vi "FFTFiltered.vi"(0 "E4S":dbl[](array[numeric]), 1 "E3S":dbl[](array[numeric]), 4 "E2S":dbl[](array[numeric]), 5 "E1S":dbl[](array[numeric]), 6 "E6S":dbl[](array[numeric]), 7 "E5S":dbl[](array[numeric]), 11 "E8S":dbl[](array[numeric]), 12 "E7S":dbl[](array[numeric]), 14 "E9S":dbl[](array[numeric]), 19 "Corte Alto":dbl(knob) scale=1.0..45.0) -> (2 "FFT X2":cluster{dbl, dbl, dbl[]}(graph), 3 "FFT X3":cluster{dbl, dbl, dbl[]}(graph), 8 "FFT X4":cluster{dbl, dbl, dbl[]}(graph), 9 "FFT X6":cluster{dbl, dbl, dbl[]}(graph), 10 "FFT X5":cluster{dbl, dbl, dbl[]}(graph), 13 "FFT X7":cluster{dbl, dbl, dbl[]}(graph), 15 "FFT X1":cluster{dbl, dbl, dbl[]}(graph), 16 "FFT X8":cluster{dbl, dbl, dbl[]}(graph), 17 "FFT X9":cluster{dbl, dbl, dbl[]}(graph))   [LabVIEW 2021]
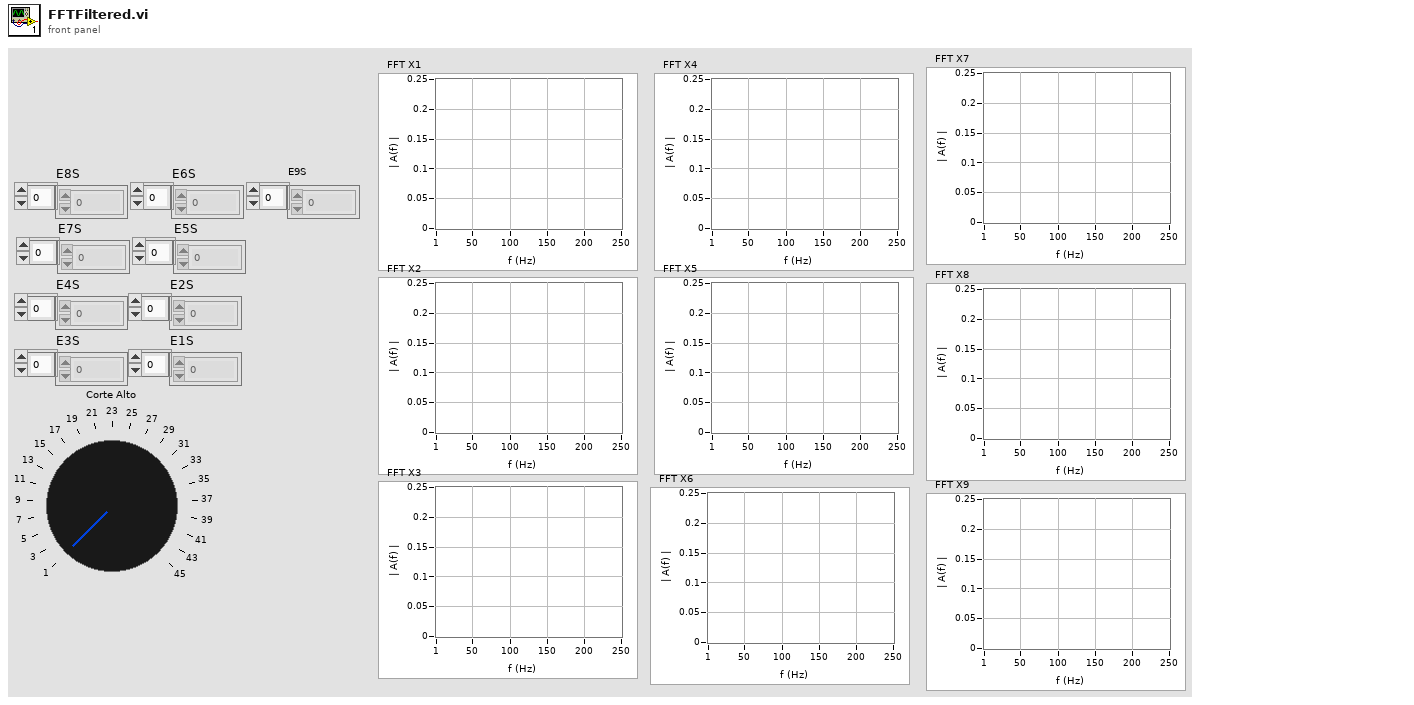
[diagram p1: front panel]
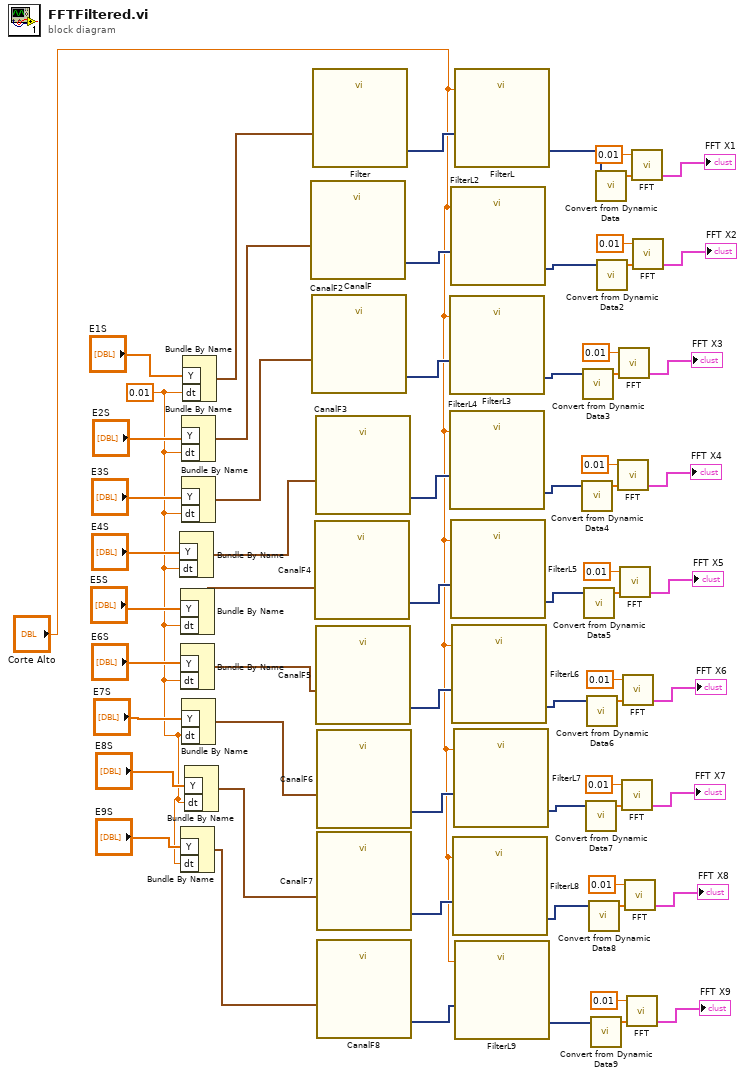
[diagram p0: block diagram]
diagram:
  w56 = 0.01 ("dt")
  n1 = Bundle By Name("Y"="E4S", "dt"=w56) -> (w52:waveform(dbl))  [unwired: 1 in]
  n2 = Bundle By Name("Y"="E5S", "dt"=w56) -> (w51:waveform(dbl))  [unwired: 1 in]
  n3 = Bundle By Name("Y"="E6S", "dt"=w56) -> (w50:waveform(dbl))  [unwired: 1 in]
  n4 = Bundle By Name("Y"="E9S", "dt"=w56) -> (w47:waveform(dbl))  [unwired: 1 in]
  n5 = Bundle By Name("Y"="E2S", "dt"=w56) -> (w54:waveform(dbl))  [unwired: 1 in]
  n6 = Bundle By Name("Y"="E3S", "dt"=w56) -> (w53:waveform(dbl))  [unwired: 1 in]
  n7 = Bundle By Name("Y"="E7S", "dt"=w56) -> (w49:waveform(dbl))  [unwired: 1 in]
  n8 = Bundle By Name("Y"="E1S", "dt"=w56) -> (w55:waveform(dbl))  [unwired: 1 in]
  n9 = Bundle By Name("Y"="E8S", "dt"=w56) -> (w48:waveform(dbl))  [unwired: 1 in]
  n10 = call "CanalF"("Signal"=w54) -> ("Filtered Signal"=w45:dynamicdata)  [unwired: 9 in, 1 out]
  n11 = call "CanalF2"("Signal"=w53) -> ("Filtered Signal"=w44:dynamicdata)  [unwired: 9 in, 1 out]
  n12 = call "Filter"("Signal"=w55) -> ("Filtered Signal"=w46:dynamicdata)  [unwired: 9 in, 1 out]
  n13 = call "CanalF4"("Signal"=w51) -> ("Filtered Signal"=w42:dynamicdata)  [unwired: 9 in, 1 out]
  n14 = call "CanalF3"("Signal"=w52) -> ("Filtered Signal"=w43:dynamicdata)  [unwired: 9 in, 1 out]
  n15 = call "CanalF5"("Signal"=w50) -> ("Filtered Signal"=w41:dynamicdata)  [unwired: 9 in, 1 out]
  n16 = call "CanalF6"("Signal"=w49) -> ("Filtered Signal"=w40:dynamicdata)  [unwired: 9 in, 1 out]
  n17 = call "CanalF7"("Signal"=w48) -> ("Filtered Signal"=w39:dynamicdata)  [unwired: 9 in, 1 out]
  n18 = call "CanalF8"("Signal"=w47) -> ("Filtered Signal"=w38:dynamicdata)  [unwired: 9 in, 1 out]
  n19 = call "FilterL3"("Lower Cut-Off"="Corte Alto", "Signal"=w44) -> ("Filtered Signal"=w7:dynamicdata)  [unwired: 8 in, 1 out]
  n20 = call "FilterL4"("Lower Cut-Off"="Corte Alto", "Signal"=w43) -> ("Filtered Signal"=w6:dynamicdata)  [unwired: 8 in, 1 out]
  n21 = call "FilterL2"("Lower Cut-Off"="Corte Alto", "Signal"=w45) -> ("Filtered Signal"=w29:dynamicdata)  [unwired: 8 in, 1 out]
  n22 = call "FilterL5"("Lower Cut-Off"="Corte Alto", "Signal"=w42) -> ("Filtered Signal"=w5:dynamicdata)  [unwired: 8 in, 1 out]
  n23 = call "FilterL6"("Lower Cut-Off"="Corte Alto", "Signal"=w41) -> ("Filtered Signal"=w4:dynamicdata)  [unwired: 8 in, 1 out]
  n24 = call "FilterL8"("Lower Cut-Off"="Corte Alto", "Signal"=w39) -> ("Filtered Signal"=w2:dynamicdata)  [unwired: 8 in, 1 out]
  n25 = call "FilterL7"("Lower Cut-Off"="Corte Alto", "Signal"=w40) -> ("Filtered Signal"=w3:dynamicdata)  [unwired: 8 in, 1 out]
  n26 = call "FilterL"("Lower Cut-Off"="Corte Alto", "Signal"=w46) -> ("Filtered Signal"=w36:dynamicdata)  [unwired: 8 in, 1 out]
  n27 = call "FilterL9"("Lower Cut-Off"="Corte Alto", "Signal"=w38) -> ("Filtered Signal"=w1:dynamicdata)  [unwired: 8 in, 1 out]
  n28 = call "Convert from Dynamic Data4"("Dynamic Data Type"=w6) -> ("Array"=w25:dbl[])  [unwired: 3 in]
  n29 = call "Convert from Dynamic Data3"("Dynamic Data Type"=w7) -> ("Array"=w28:dbl[])  [unwired: 3 in]
  n30 = call "Convert from Dynamic Data5"("Dynamic Data Type"=w5) -> ("Array"=w22:dbl[])  [unwired: 3 in]
  n31 = call "Convert from Dynamic Data7"("Dynamic Data Type"=w3) -> ("Array"=w16:dbl[])  [unwired: 3 in]
  n32 = call "Convert from Dynamic Data6"("Dynamic Data Type"=w4) -> ("Array"=w19:dbl[])  [unwired: 3 in]
  n33 = call "Convert from Dynamic Data8"("Dynamic Data Type"=w2) -> ("Array"=w13:dbl[])  [unwired: 3 in]
  n34 = call "Convert from Dynamic Data9"("Dynamic Data Type"=w1) -> ("Array"=w10:dbl[])  [unwired: 3 in]
  n35 = call "Convert from Dynamic Data"("Dynamic Data Type"=w36) -> ("Array"=w35:dbl[])  [unwired: 3 in]
  n36 = call "Convert from Dynamic Data2"("Dynamic Data Type"=w29) -> ("Array"=w32:dbl[])  [unwired: 3 in]
  n37 = call "FFT.vi"("Y"=w25, "dt"=0.01) -> ("FFT Señal"=→"FFT X4":cluster{dbl, dbl, dbl[]})  [unwired: 1 in, 2 out]
  n38 = call "FFT.vi"("Y"=w28, "dt"=0.01) -> ("FFT Señal"=→"FFT X3":cluster{dbl, dbl, dbl[]})  [unwired: 1 in, 2 out]
  n39 = call "FFT.vi"("Y"=w22, "dt"=0.01) -> ("FFT Señal"=→"FFT X5":cluster{dbl, dbl, dbl[]})  [unwired: 1 in, 2 out]
  n40 = call "FFT.vi"("Y"=w16, "dt"=0.01) -> ("FFT Señal"=→"FFT X7":cluster{dbl, dbl, dbl[]})  [unwired: 1 in, 2 out]
  n41 = call "FFT.vi"("Y"=w19, "dt"=0.01) -> ("FFT Señal"=→"FFT X6":cluster{dbl, dbl, dbl[]})  [unwired: 1 in, 2 out]
  n42 = call "FFT.vi"("Y"=w13, "dt"=0.01) -> ("FFT Señal"=→"FFT X8":cluster{dbl, dbl, dbl[]})  [unwired: 1 in, 2 out]
  n43 = call "FFT.vi"("Y"=w10, "dt"=0.01) -> ("FFT Señal"=→"FFT X9":cluster{dbl, dbl, dbl[]})  [unwired: 1 in, 2 out]
  n44 = call "FFT.vi"("Y"=w35, "dt"=0.01) -> ("FFT Señal"=→"FFT X1":cluster{dbl, dbl, dbl[]})  [unwired: 1 in, 2 out]
  n45 = call "FFT.vi"("Y"=w32, "dt"=0.01) -> ("FFT Señal"=→"FFT X2":cluster{dbl, dbl, dbl[]})  [unwired: 1 in, 2 out]
